vi "Initialize Passwords.vi"(8 "error in (no error)":errorcluster) -> (0 "error out":errorcluster, 2 "Access Configuration":T1 {"User array"."Expire sec" format="%.2f"}, 3 "dup path":path)   [LabVIEW 2013]
doc: "Initializes the Password modules. If no file is found a new password file is generated with a single user \nUser name:admin\nPW: admin\nsecurity level:10"
uses:
  User Access Type defs/Security level U8.ctl
  User Access Type defs/User access cluster.ctl
  User Access Type defs/User access cluster array.ctl
  User Access Type defs/All users access configuration cluster.ctl
  Host/File IO/File Paths Global.vi
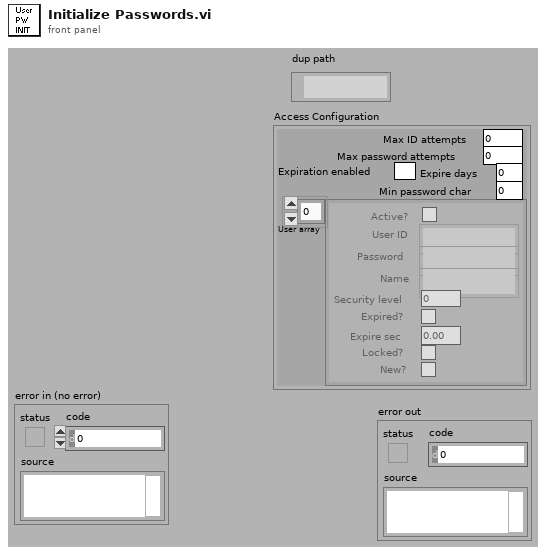
[diagram p1: front panel]
types:
  T1 = typedef "All users access configuration cluster.ctl" = cluster{"Max ID attempts":i32, "Max password attempts":i32, "Expiration enabled":bool, "Expire days":i32, "User array":T2, "Min password char":i32}
  T2 = typedef "User access cluster array.ctl" = T3[]
  T3 = typedef "User access cluster.ctl" = cluster{"Active?":bool, "User ID":string, "Password":string, "Name":string, "Security level":T4, "Expired?":bool, "Expire sec":dbl, "Locked?":bool, "New?":bool}
  T4 = typedef "Security level U8.ctl" = u8
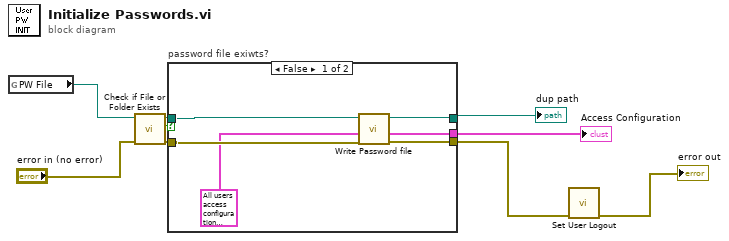
[diagram p0: block diagram]
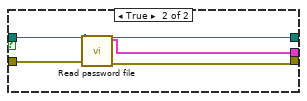
[diagram p2: hidden frame]
diagram:
  n1 = global read "File Paths Global.vi" "PW File"() -> (w1:path)
  n2 = call <vilib>:"Check if File or Folder Exists.vi"("error in (no error)"="error in (no error)", "path"=w1) -> ("error out"=w5:errorcluster, "file or folder exists?"=w8:bool, "dup path"=w6:path)  [unwired: 7 out]
  n3 = case "password file exiwts?" shown="False" w8 {
    tunnel: w5 -> [w13 w17]
    tunnel: w6 -> [w10 w14]
    tunnel: [w12 w15] -> w4
    tunnel: [w11 w16] -> w2
    tunnel: [w10 w14] -> w9
    frame False {
      w12 = T1 {"Max ID attempts"=3, "Max password attempts"=4, "Expiration enabled"=FALSE, "Expire days"=90, "User array"=[{"Active?"=TRUE, "User ID"="Admin", "Password"="admin", "Name"="Administrator", "Security level"=10, "Expired?"=FALSE, "Expire sec"=inf, "Locked?"=FALSE, "New?"=FALSE}], "Min password char"=5} ("Access Configuration")
      n4 = call "Write Password file.vi"("error in (no error)"=w13, "Access Configuration"=w12, "Path"=w10) -> ("error out"=w11:errorcluster)  [unwired: 8 out]
    }
    frame True {
      n5 = call "Read password file.vi"("error in (no error)"=w17, "file path"=w14) -> ("error out"=w16:errorcluster, "Access Configuration"=w15:T1)  [unwired: 8 out]
    }
  }
  "dup path" <- w9
  "Access Configuration" <- w4
  n6 = call "Set User Logout.vi"("error in"=w2) -> ("error out"=→"error out":errorcluster)  [unwired: 10 out]
